vi "External Acturator Volts 2 Readings.vi"(10 "Settings":T1(array[cluster]), 11 "External Actuator Volts In":dbl[](array[numeric])) -> (3 "External Actuator Readings Out":dbl[](array[numeric]))   [LabVIEW 2009]
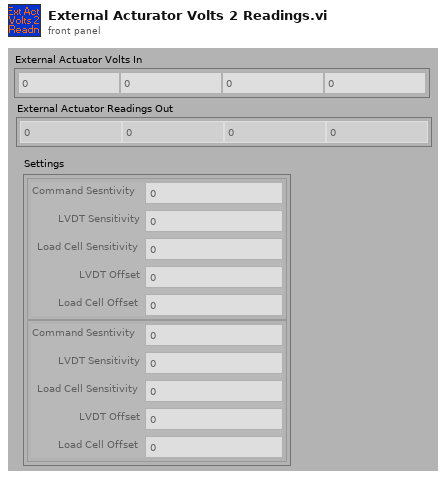
[diagram p1: front panel]
types:
  T1 = cluster{"Load Cell Sensitivity":dbl, "Command Sesntivity":dbl, "LVDT Sensitivity":dbl, "LVDT Offset":dbl, "Load Cell Offset":dbl}[]
  T2 = cluster{"Load Cell Sensitivity":dbl, "Command Sesntivity":dbl, "LVDT Sensitivity":dbl, "LVDT Offset":dbl, "Load Cell Offset":dbl}
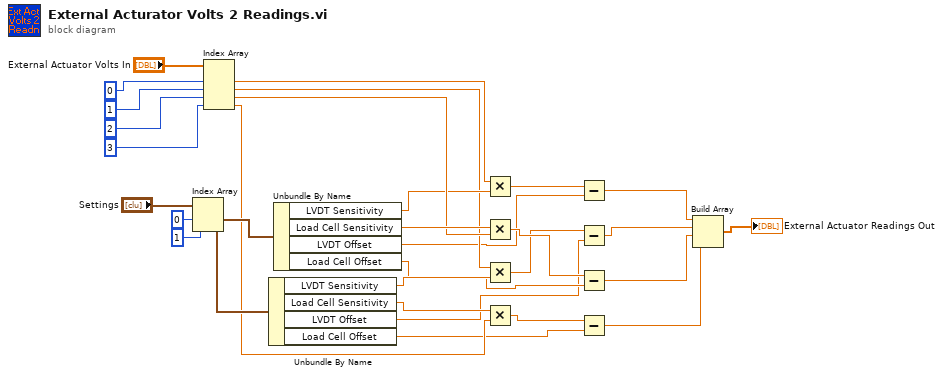
[diagram p0: block diagram]
diagram:
  n1 = Index Array(array="Settings", index #1=0 ("index"), index #2=1 ("index")) -> (element #1=w23:T2, element #2=w18:T2)
  n2 = Index Array(array="External Actuator Volts In", index #1=0 ("index"), index #2=1 ("index"), index #3=2 ("index"), index #4=3 ("index")) -> (element #1=w15:dbl, element #2=w12:dbl, element #3=w21:dbl, element #4=w17:dbl)
  n3 = Unbundle By Name(w18) -> ("LVDT Sensitivity"=w11:dbl, "Load Cell Sensitivity"=w19:dbl, "LVDT Offset"=w4:dbl, "Load Cell Offset"=w1:dbl)
  n4 = Unbundle By Name(w23) -> ("LVDT Sensitivity"=w14:dbl, "Load Cell Sensitivity"=w22:dbl, "LVDT Offset"=w9:dbl, "Load Cell Offset"=w7:dbl)
  n5 = Multiply(x=w15, y=w14) -> (x*y=w13:dbl)
  n6 = Multiply(x=w22, y=w21) -> (x*y=w20:dbl)
  n7 = Multiply(x=w12, y=w11) -> (x*y=w5:dbl)
  n8 = Multiply(x=w19, y=w17) -> (x*y=w2:dbl)
  n9 = Subtract(x=w13, y=w9) -> (x-y=w10:dbl)
  n10 = Subtract(x=w5, y=w4) -> (x-y=w6:dbl)
  n11 = Subtract(x=w20, y=w7) -> (x-y=w8:dbl)
  n12 = Subtract(x=w2, y=w1) -> (x-y=w3:dbl)
  n13 = Build Array(w10, w6, w8, w3) -> (→"External Actuator Readings Out":dbl[])
